vi "Z900_navX_SPI_Read.vi"(8 "error in (no error)":errorcluster, 10 "Registry":u8[](array[numeric]), 11 "Interface TypeDefs":T1 {"I2CDevRef"."Device Address" format="%.0x"}) -> (0 "error out":errorcluster, 1 "Valid":bool, 2 "Registry":u8[](array[numeric]), 3 "Interface TypeDefs":T1 {"I2CDevRef"."Device Address" format="%.0x"})   [LabVIEW 2015, in "navX Library v2.lvlib"]
uses:
  navX Library v2.lvlib
  _TypeDefs/Z900_navX_InterfaceTypeDef.ctl
  <vilib>/Rock Robotics/WPI/SerialPort/WPI_SerialPortRef.ctl
  <vilib>/Rock Robotics/WPI/I2C/WPI_I2CDevRef.ctl
  <vilib>/Rock Robotics/SystemInterfaces/i2clib/i2c_bus.ctl
  <vilib>/Rock Robotics/WPI/SPI/WPI_SPIDevRef.ctl
  <vilib>/Rock Robotics/SystemInterfaces/spilib/spi_bus.ctl
  _TypeDefs/Z900_navX_DeviceRegisters.ctl
  _TypeDefs/Flags/Z900_navX_Flags_CapabilityTypeDef.ctl
  _Util/Z900_navX_Util_LittleEndian_to_BigEndian.vi
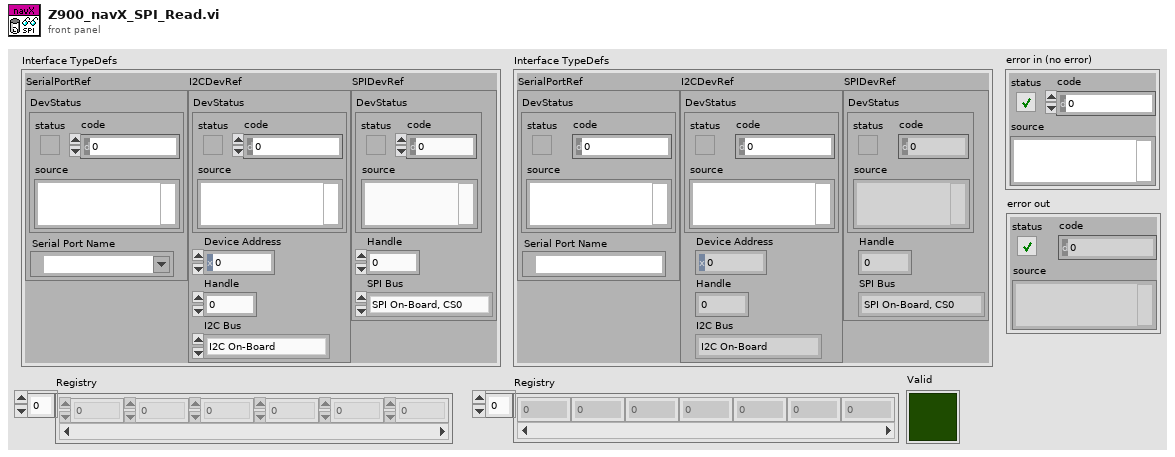
[diagram p1: front panel]
types:
  T1 = typedef "navX Library v2.lvlib/Z900_navX_InterfaceTypeDef.ctl" = cluster{"SerialPortRef":T2, "I2CDevRef":T3, "SPIDevRef":T5}
  T2 = typedef "WPI_SerialPortRef.ctl" = cluster{"DevStatus":errorcluster, "Serial Port Name":refnum<visa-resource-name>}
  T3 = typedef "WPI_I2CDevRef.ctl" = cluster{"DevStatus":errorcluster, "Device Address":u8, "Handle":i32, "I2C Bus":T4}
  T4 = typedef "i2c_bus.ctl" = enum16{"I2C On-Board", "I2C MXP", "Invalid"}
  T5 = typedef "WPI_SPIDevRef.ctl" = cluster{"DevStatus":errorcluster, "Handle":i32, "SPI Bus":T6}
  T6 = typedef "spi_bus.ctl" = enum16{"SPI On-Board, CS0", "SPI On-Board, CS1", "SPI On-Board, CS2", "SPI On-Board, CS3", "SPI MXP", "Invalid"}
  T7 = typedef "navX Library v2.lvlib/Z900_navX_Flags_CapabilityTypeDef.ctl" = u16
  T8 = typedef "navX Library v2.lvlib/Z900_navX_DeviceRegisters.ctl" = u8
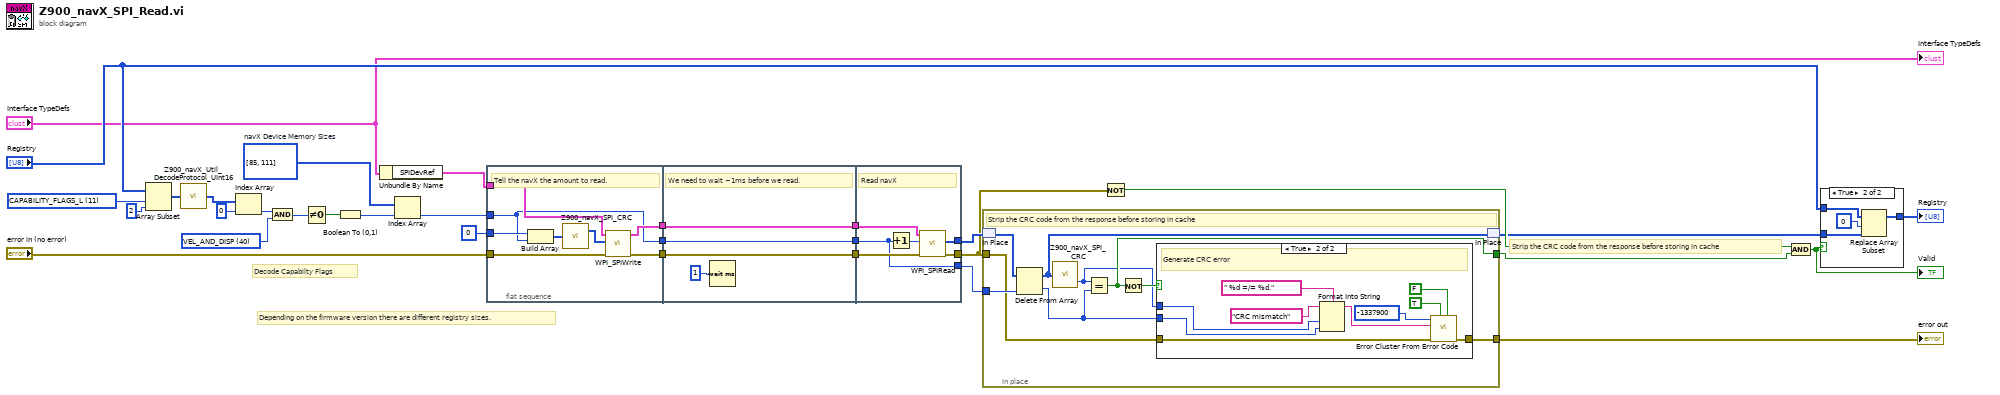
[diagram p0: block diagram]
diagram:
  w10 = T7 40 items=["OMNIMOUNT"=4, "OMNIMOUNT_CONFIG_MASK"=38, "VEL_AND_DISP"=40, "YAW_RESET"=80] ("Capability Flag")
  w12 = T8 11 items=["WHOAMI"=0, "HW_REV"=1, "FW_VER_MAJOR"=2, "FW_VER_MINOR"=3, "UPDATE_RATE_HZ"=4, "ACCEL_FSR_G"=5, "GYRO_FSR_DPS"=6, "OP_STATUS"=8, "CAL_STATUS"=9, "SELFTEST_STATUS"=10, "CAPABILITY_FLAGS_L"=11, "CAPABILITY_FLAGS_H"=12, "SENSOR_STATUS"=16, "TIMESTAMP"=18, "YAW"=22, "ROLL"=24, "PITCH"=26, "HEADING"=28, "FUSED_HEADING"=30, "ALTITUDE_I"=32, "ALTITUDE_D"=34, "LINERA_ACC_X"=36, "LINERA_ACC_Y"=38, "LINERA_ACC_Z"=40, "QUAT_W"=42, "QUAT_X"=44, "QUAT_Y"=46, "QUAT_Z"=48, "MPU_TEMP_C"=50, "GYRO_X"=52, "GYRO_Y"=54, "GYRO_Z"=56, "ACC_X"=58, "ACC_Y"=60, "ACC_Z"=62, "MAG_X"=64, "MAG_Y"=66, "MAG_Z"=68, "PRESSURE_I"=70, "PRESSURE_D"=72, "PRESSURE_TEMP"=74, "YAW_OFFSET"=76, "QUAT_OFFSET_W"=78, "QUAT_OFFSET_X"=80, "QUAT_OFFSET_Y"=82, "QUAT_OFFSET_Z"=84, "INTEGRATION_CONTROL"=86, "VELOCITY_X"=88, "VELOCITY_Y"=92, "VELOCITY_Z"=96, "DISPLACMENT_X"=100, "DISPLACMENT_Y"=104, "DISPLACEMENT_Z"=108] ("Device Register")
  w23 = i32[] [85, 111]  # navX Device Memory Sizes
  # "Strip the CRC code from the response before storing in cache"
  # "Decode Capabilty Flags"
  # "Depending on the firmware version there are different registry sizes."
  n1 = Array Subset(array="Registry", index=w12, length=2) -> (w16:u8[])
  n2 = call "Z900_navX_Util_DecodeProtocol_UInt16.vi"("Little Endian"=w16) -> ("UInt16"=w17:u16[])
  n3 = Index Array(array=w17, index=0) -> (element=w15:u16)
  n4 = And(x=w15, y=w10) -> (x .and. y?=w9:T7)
  n5 = Not Equal To 0?(x=w9) -> (x != 0?=w14:bool)
  n6 = Boolean To (0,1)(Boolean=w14) -> (0, 1=w13:i16)
  n7 = Unbundle By Name("Interface TypeDefs") -> ("SPIDevRef"=w25:T5)
  n8 = Index Array(array=w23, index=w13) -> (element=w24:i32)
  n9 = flat-sequence {
    tunnel: u8 0 ("hex") -> [w40]
    tunnel: w24 -> [w35]
    tunnel: w25 -> [w37]
    tunnel: [w36] -> w32
    tunnel: [w35] -> w31
    tunnel: [w34] -> w30
    tunnel: "error in (no error)" -> [w33]
    tunnel: w32 -> [w43]
    tunnel: [w43] -> w29
    tunnel: [w42] -> w28
    tunnel: w31 -> [w42]
    tunnel: w30 -> [w41]
    tunnel: [w41] -> w27
    tunnel: [w45] -> w4
    tunnel: [w46] -> w5
    tunnel: [w47] -> w6
    tunnel: w27 -> [w48]
    tunnel: w28 -> [w46]
    tunnel: w29 -> [w50]
    frame #0 {
      # "Tell the navX the amount to read."
      n10 = Build Array(w40, w35) -> (w39:i32[])
      n11 = call "Z900_navX_SPI_CRC.vi"("Message"=w39) -> ("Message with CRC"=w38:u8[])  [unwired: 1 out]
      n12 = call <vilib>:"WPI_SPIWrite.vi"("error in (no error)"=w33, "Data To Send"=w38, "SPIDevRef"=w37) -> ("error out"=w34:errorcluster, "SPIDevRef"=w36:T5)  [unwired: 6 in, 1 out]
    }
    frame #1 {
      # "We need to wait ~1ms before we read."
      n13 = Wait (ms)(milliseconds to wait=u32 1) -> ()  [unwired: 1 out]
    }
    frame #2 {
      # "Read navX"
      n14 = Increment(x=w46) -> (x+1=w49:i32)
      n15 = call <vilib>:"WPI_SPIRead.vi"("error in (no error)"=w48, "Num to Read"=w49, "SPIDevRef"=w50) -> ("error out"=w45:errorcluster, "Received Data"=w47:u8[])  [unwired: 6 in, 1 out]
    }
  }
  n16 = in-place {
    in-place-border: w5 -> [w59]
    in-place-border: [w56] -> w7
    in-place-border: w4 -> [w52]
    in-place-border: [w51] -> w1
    # "Strip the CRC code from the response before storing in cache"
    n17 = in-place-match #1(w6) -> (w58:u8[])
    n18 = Delete From Array(array=w58, index=w59) -> (deleted portion=w53:u8, array with subset deleted=w57:u8[])  [unwired: 1 in]
    n19 = call "Z900_navX_SPI_CRC.vi"("Message"=w57) -> ("CRC"=w54:u8)  [unwired: 1 out]
    n20 = Equal?(x=w54, y=w53) -> (x = y?=w56:bool)
    n21 = Not(x=w56) -> (.not. x?=w55:bool)
    n22 = case shown="True" w55 {
      tunnel: w54 -> [_ w68]
      tunnel: w53 -> [_ w67]
      tunnel: w52 -> [w60 w64]
      tunnel: [w60 w63] -> w51
      frame False {
      }
      frame True {
        # "Generate CRC error"
        n23 = Format Into String(format string=" %d =/= %d.", initial string="CRC mismatch", w68, w67) -> (resulting string=w65:string)  [unwired: 1 in, 1 out]
        n24 = call <vilib>:"Error Cluster From Error Code.vi"("is warning? (False)"=FALSE, "show call chain? (False)"=TRUE, "error in (no error)"=w64, "error message (\"\")"=w65, "error code (0)"=-1337900 ("code")) -> ("error out"=w63:errorcluster)  [unwired: 4 in]
      }
    }
    n25 = in-place-match #1(w57) -> (w3:u8[])
  }
  "error out" <- w1
  n26 = Not(x=w4) -> (.not. x?=w8:bool)
  n27 = And(x=w8, y=w7) -> (x .and. y?=w2:bool)
  "Valid" <- w2
  n28 = case shown="True" w2 {
    tunnel: "Registry" -> [w71 w75]
    tunnel: [w71 w74] -> w21
    tunnel: w3 -> [_ w73]
    frame False {
    }
    frame True {
      n29 = Replace Array Subset(array=w75, new element=w73, index=u8 0 ("hex")) -> (w74:u8[])
    }
  }
  "Registry" <- w21
  "Interface TypeDefs" <- "Interface TypeDefs"
